vi "Read Iterator Shift.vi"(11 "Circular Buffer in":refnum<class "Circular Buffer.lvclass">) -> (2 "shift":i64, 3 "Circular Buffer out":refnum<class "Circular Buffer.lvclass">)   [LabVIEW 2021, in "d20.lvlib" / "Circular Buffer.lvclass"]
uses:
  Circular Buffer.lvclass
  Circular Buffer.lvclass/Circular Buffer.ctl
  INode/INode.lvclass
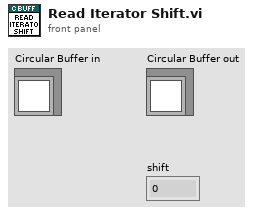
[diagram p1: front panel]
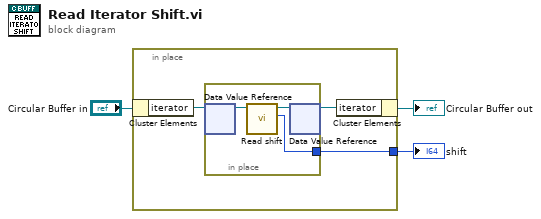
[diagram p0: block diagram]
diagram:
  n1 = in-place {
    in-place-border: [w5] -> w1
    n2 = in-place-cluster #1("Circular Buffer in") -> ("iterator"=w6:refnum<data-value>)
    n3 = in-place {
      in-place-border: [w9] -> w5
      n4 = in-place-dvr #2(w6) -> (w7:refnum<class "INode.lvclass">)  [unwired: 1 out]
      n5 = call-dynamic "Read shift.vi"("Node in"=w7) -> ("shift"=w9:i64, "Node out"=w8:refnum<class "INode.lvclass">)  [unwired: 9 in]
      n6 = in-place-dvr #2(w8) -> (w4:refnum<data-value>)  [unwired: 1 out]
    }
    n7 = in-place-cluster #1("iterator"=w4) -> (→"Circular Buffer out":refnum<class "Circular Buffer.lvclass">)
  }
  "shift" <- w1
